vi "FGV Ventile Vis Komm.vi"(0 "Ventile schalten":u32, 7 "Betrieb":u16, 11 "error in (no error)":errorcluster caption="Fehler (Eingang, kein Fehler)", 13 "Aktion":enum16{"lesen", "schreiben"}(ring)) -> (4 "Ventile schalten":u32, 8 "Betrieb":u16, 15 "error out":errorcluster caption="Fehler (Ausgang)")   [LabVIEW 2020, in "Allgemein.lvlib"]
uses:
  Allgemein.lvlib
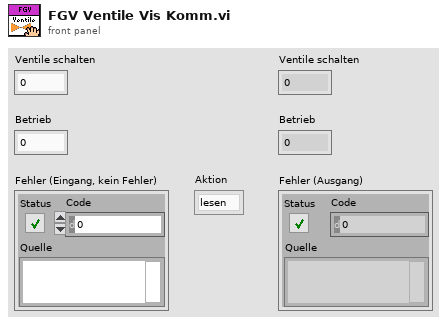
[diagram p1: front panel]
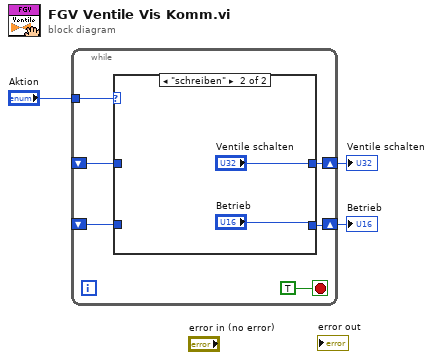
[diagram p0: block diagram]
diagram:
  n1 = while {
    tunnel: "Aktion" -> [w8]
    shift-right: [w7] -> w2
    shift-left: _ -> [w6]
    shift-right: [w5] -> w1
    shift-left: _ -> [w4]
    stop <- TRUE stop-if-true
    n2 = case shown="\"schreiben\"" w8 {
      tunnel: [w11 "Ventile schalten"] -> w7
      tunnel: w6 -> [w11 _]
      tunnel: [w10 "Betrieb"] -> w5
      tunnel: w4 -> [w10 _]
      frame "lesen", Default {
      }
      frame "schreiben" {
      }
    }
  }
  "Ventile schalten" <- w2
  "Betrieb" <- w1
